vi "Validate Query Input.vi"(9 "Timeout (s)":dbl=15.0, 11 "Query in":string) -> (1 "Timeout (ms)":i32, 2 "Call Procedure?":bool, 3 "Query out":string)   [LabVIEW 2014, in "hse-db.lvlib" / "MySQL (TCP).lvlib"]
uses:
  MySQL (TCP).lvlib
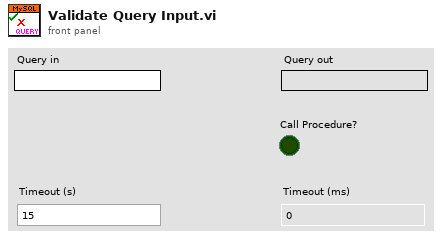
[diagram p1: front panel]
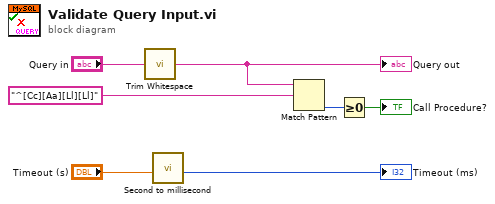
[diagram p0: block diagram]
diagram:
  n1 = call <vilib>:"Trim Whitespace.vi"("string"="Query in") -> ("trimmed string"=w5:string)  [unwired: 1 in]
  "Query out" <- w5
  n2 = call "Second to millisecond.vi"("Timeout"="Timeout (s)") -> ("Timeout (ms)"=→"Timeout (ms)":i32)  [unwired: 10 in]
  n3 = Match Pattern(string=w5, regular expression="^[Cc][Aa][Ll][Ll]") -> (offset past match=w4:i32)  [unwired: 1 in, 3 out]
  n4 = Greater Or Equal To 0?(x=w4) -> (x >= 0?=→"Call Procedure?":bool)
